vi "Actualizar monedas.vi"(6 "wait for reply (T)":bool=TRUE, 8 "error in (no error)":errorcluster) -> (0 "error out":errorcluster, 1 "timed out?":bool, 3 "Reply Payload":T1)   [LabVIEW 2020]
doc: "Actualiza la denominaciónd e cada una de las monedas y si es visible o no\n_____\nCreated using Delacor QMH Event Scripter 5.0.0.112."
uses:
  Actualizar monedas Argument--cluster.ctl
  Actualizar monedas (Reply Payload)--cluster.ctl
  Config.lvlib
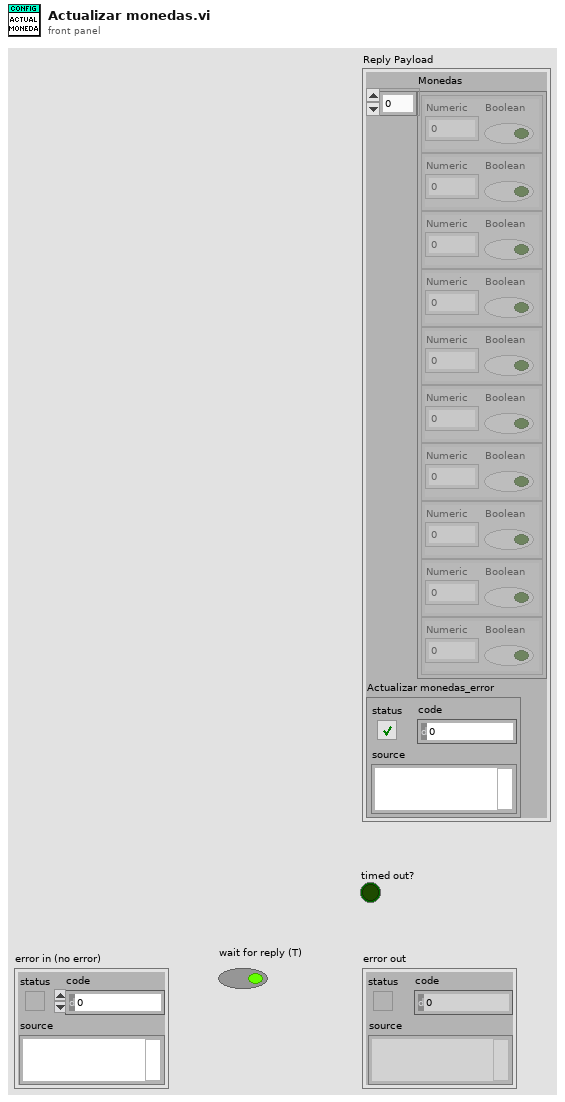
[diagram p1: front panel]
types:
  T1 = typedef "Actualizar monedas (Reply Payload)--cluster.ctl" = cluster{"Monedas":cluster{"Numeric":dbl, "Boolean":bool}[], "Actualizar monedas_error":errorcluster}
  T2 = typedef "Actualizar monedas Argument--cluster.ctl" = cluster{"Wait Notifier":refnum<notifier>, "wait for reply":bool}
  T3 = typedef "Config.lvlib/Request Events--cluster.ctl" = cluster{"Stop Module":refnum<user-event>, "Show Panel":refnum<user-event>, "Hide Panel":refnum<user-event>, "Get Module Execution Status":refnum<user-event>, "Show Diagram":refnum<user-event>}
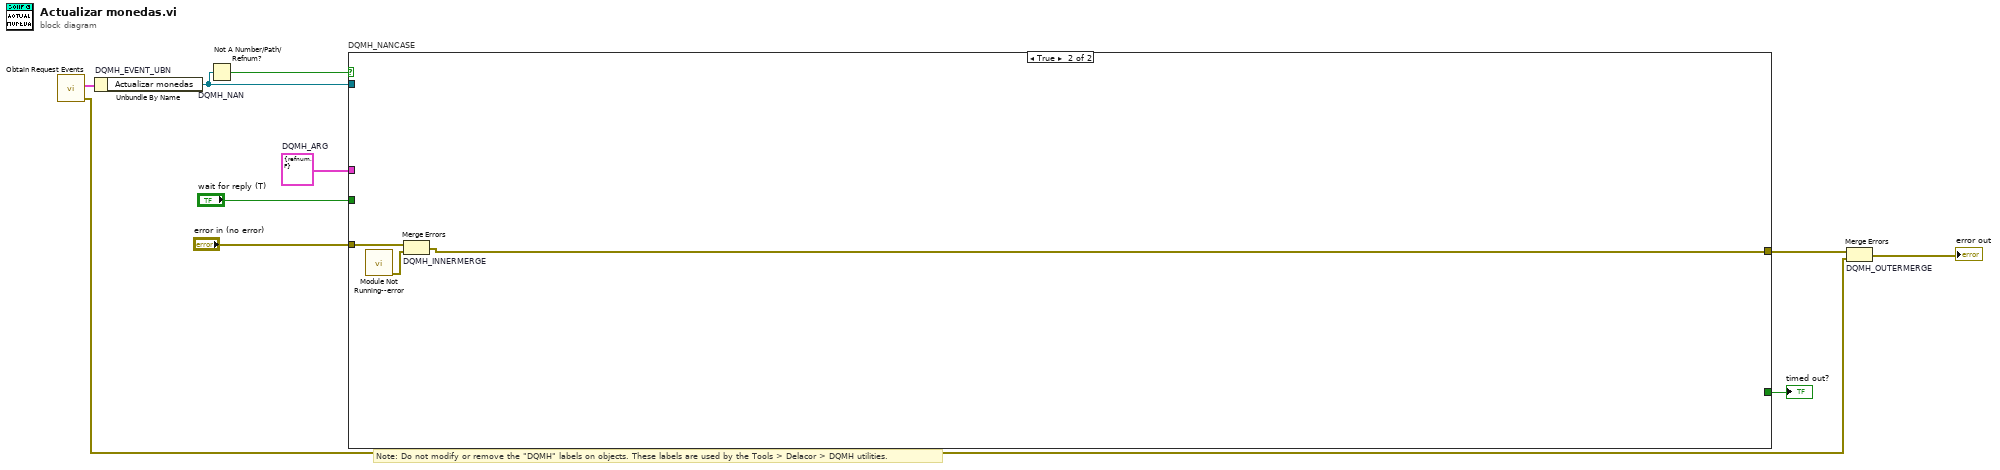
[diagram p0: block diagram]
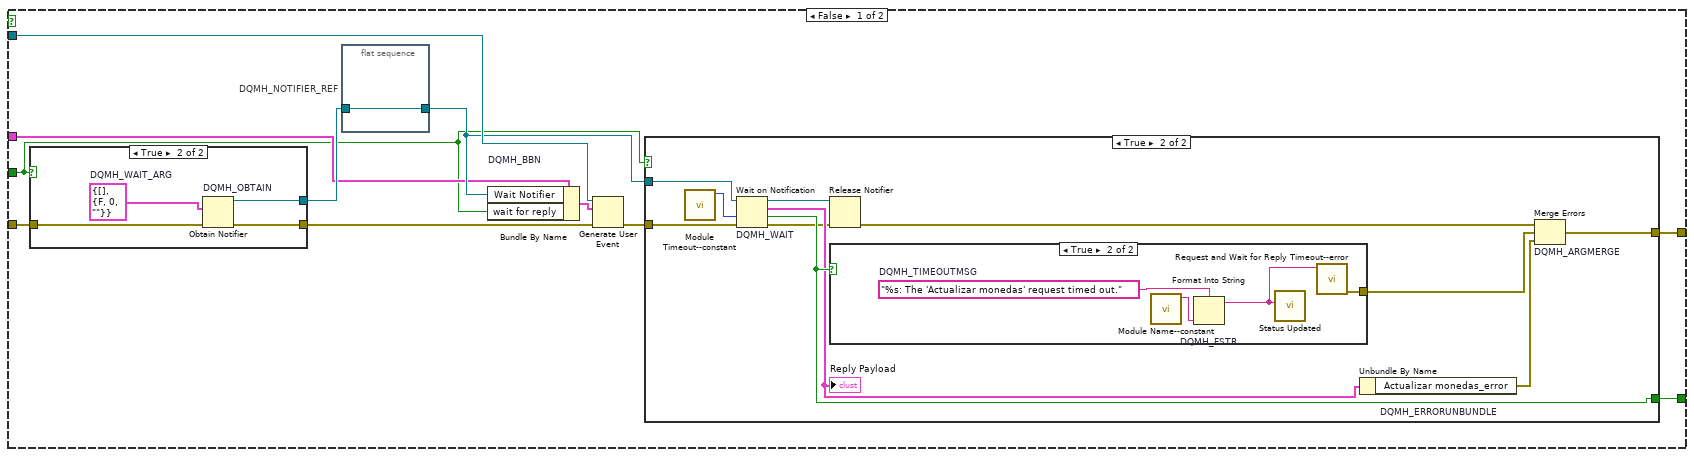
[diagram p2: hidden frame]
diagram:
  w4 = T2 {"Wait Notifier"=refnum, "wait for reply"=FALSE}  # DQMH_ARG
  # "Note: Do not modify or remove the \"DQMH\" labels on objects. These labels are used by the Tools > Delacor > DQMH utilities."
  n1 = call "Obtain Request Events.vi"() -> ("error out"=w2:errorcluster, "Config Request Events"=w1:T3)  [unwired: 10 in]
  n2 = Unbundle By Name "DQMH_EVENT_UBN"(w1) -> ("Actualizar monedas"=w8:refnum<user-event>)
  n3 = Not A Number/Path/Refnum? "DQMH_NAN"(number/path/refnum=w8) -> (NaN/Path/Refnum?=w7:bool)
  n4 = case "DQMH_NANCASE" shown="True" w7 {
    tunnel: "error in (no error)" -> [w21 w46]
    tunnel: w8 -> [w19 _]
    tunnel: [w16 w45] -> w5
    tunnel: [w17 _] -> w6
    tunnel: w4 -> [w12 _]
    tunnel: "wait for reply (T)" -> [w11 _]
    frame False {
      n5 = case shown="True" w11 {
        tunnel: w21 -> [w39 w43]
        tunnel: [w39 w42] -> w18
        tunnel: [_ w40] -> w14
        frame False {
        }
        frame True {
          w41 = T1 {"Monedas"=[], "Actualizar monedas_error"={"status"=FALSE, "code"=0, "source"=""}}  # DQMH_WAIT_ARG
          n6 = Obtain Notifier "DQMH_OBTAIN"(notification data type=w41, error in (no error)=w43) -> (notifier out=w40:refnum<notifier>, error out=w42:errorcluster)  [unwired: 2 in, 1 out]
        }
      }
      n7 = flat-sequence "DQMH_NOTIFIER_REF" {
        tunnel: w14 -> [w22]
        tunnel: [w22] -> w13
        frame #0 {
        }
      }
      n8 = Bundle By Name "DQMH_BBN"(cluster=w12, "Wait Notifier"=w13, "wait for reply"=w11) -> (w15:T2)
      n9 = Generate User Event(user event=w19, event data cluster=w15, error in=w18) -> (error out=w20:errorcluster)  [unwired: 1 in, 1 out]
      n10 = case shown="True" w11 {
        tunnel: w20 -> [w23 w34]
        tunnel: w13 -> [_ w33]
        tunnel: [_ w31] -> w17
        tunnel: [w23 w30] -> w16
        frame False {
        }
        frame True {
          n11 = call "Module Timeout--constant.vi"() -> ("Module Timeout"=w24:i32)  [unwired: 11 in]
          n12 = Wait on Notification "DQMH_WAIT"(notifier=w33, timeout in ms (-1)=w24, error in (no error)=w34) -> (notifier out=w32:refnum<notifier>, notification=w29:T1, timed out?=w31:bool, error out=w28:errorcluster)  [unwired: 1 in]
          "Reply Payload" <- w29
          n13 = Release Notifier(notifier=w32, error in (no error)=w28) -> (error out=w27:errorcluster)  [unwired: 1 in, 2 out]
          n14 = case shown="True" w31 {
            tunnel: [_ w36] -> w25
            frame False {
            }
            frame True {
              w38 = "%s: The 'Actualizar monedas' request timed out."  # DQMH_TIMEOUTMSG
              n15 = call "Module Name--constant.vi"() -> ("Module Name"=w35:string)  [unwired: 11 in]
              n16 = Format Into String "DQMH_FSTR"(format string=w38, w35) -> (resulting string=w37:string)  [unwired: 2 in, 1 out]
              n17 = call "Status Updated.vi"("Status"=w37) -> ()  [unwired: 10 in, 1 out]
              n18 = call "Request and Wait for Reply Timeout--error.vi"("Error Message"=w37) -> ("error out"=w36:errorcluster)  [unwired: 10 in]
            }
          }
          n19 = Unbundle By Name "DQMH_ERRORUNBUNDLE"(w29) -> ("Actualizar monedas_error"=w26:errorcluster)
          n20 = Merge Errors "DQMH_ARGMERGE"(w27, w25, w26) -> (w30:errorcluster)
        }
      }
    }
    frame True {
      n21 = call "Module Not Running--error.vi"() -> ("error out"=w44:errorcluster)  [unwired: 11 in]
      n22 = Merge Errors "DQMH_INNERMERGE"(w46, w44) -> (w45:errorcluster)
    }
  }
  "timed out?" <- w6
  n23 = Merge Errors "DQMH_OUTERMERGE"(w5, w2) -> (→"error out":errorcluster)
